vi "delay_image_analyseR2.vi"(0 "Image File List":string[](array[string])=["spectrum26270.000msh3000usd6.500dac0atoms.bny", "spectrum26270.000msh3000usd6.500dac1atoms.bny", "spectrum26270.000msh3000usd6.500dac2atoms.bny", "spectrum26270.000msh3000usd6.500dac3atoms.bny", "spectrum26270.000msh3000usd6.500dac4atoms.bny", "spectrum26270.000msh3000usd6.500dac5atoms.bny", "spectrum26270.000msh3000usd6.500dac6atoms.bny", "spectrum26270.000msh3000usd6.500dac7atoms.bny", "spectrum26270.000msh3000usd6.500dac8atoms.bny", "spectrum26270.000msh3000usd6.500dac9atoms.bny", "spectrum26270.000msh3000usd6.500dac10atoms.bny", "spectrum26270.000msh3000usd6.500dac11atoms.bny", "spectrum26270.000msh3000usd6.500dac12atoms.bny", "spectrum26270.000msh3000usd6.500dac13atoms.bny", "spectrum26270.000msh3000usd6.500dac14atoms.bny", "spectrum26270.000msh3000usd6.500dac15atoms.bny", "spectrum26270.000msh3000usd6.500dac16atoms.bny", "spectrum26270.000msh3000usd6.500dac17atoms.bny", "spectrum26270.000msh3000usd6.500dac18atoms.bny", "spectrum26270.000msh3000usd6.500dac19atoms.bny", "spectrum26270.000msh3000usd6.500dac20atoms.bny", "spectrum26270.000msh3000usd6.500dac21atoms.bny", "spectrum26270.000msh3000usd6.500dac22atoms.bny", "spectrum26270.000msh3000usd6.500dac23atoms.bny", "spectrum26270.000msh3000usd6.500dac24atoms.bny", "spectrum26270.000msh3000usd6.500dac25atoms.bny", "spectrum26270.000msh3000usd6.500dac26atoms.bny", "spectrum26270.000msh3000usd6.500dac27atoms.bny", "spectrum26270.000msh3000usd6.500dac28atoms.bny", "spectrum26270.000msh3000usd6.500dac29atoms.bny", "spectrum26270.000msh3000usd6.500dac30atoms.bny", "spectrum26270.000msh3000usd6.500dac31atoms.bny", "spectrum26270.000msh3000usd6.500dac32atoms.bny", "spectrum26270.000msh3000usd6.500dac33atoms.bny", "spectrum26270.000msh3000usd6.500dac34atoms.bny", "spectrum26270.000msh3000usd6.500dac35atoms.bny", "spectrum26270.000msh3000usd6.500dac36atoms.bny", "spectrum26270.000msh3000usd6.500dac37atoms.bny", "spectrum26270.000msh3000usd6.500dac38atoms.bny", "spectrum26270.000msh3000usd6.500dac39atoms.bny", "spectrum26270.000msh3000usd6.500dac40atoms.bny", "spectrum26270.000msh3000usd6.500dac41atoms.bny", "spectrum26270.000msh3000usd6.500dac42atoms.bny", "spectrum26270.000msh3000usd6.500dac43atoms.bny", "spectrum26270.000msh3000usd6.500dac44atoms.bny", "spectrum26270.000msh3000usd6.500dac45atoms.bny", "spectrum26270.000msh3000usd6.500dac46atoms.bny", "spectrum26270.000msh3000usd6.500dac47atoms.bny", "spectrum26270.000msh3000usd6.500dac48atoms.bny", "spectrum26270.000msh3000usd6.500dac49atoms.bny", "spectrum26270.000msh3000usd6.500dac50atoms.bny", "spectrum26270.000msh3000usd6.500dac51atoms.bny", "spectrum26270.000msh3000usd6.500dac52atoms.bny", "spectrum26270.000msh3000usd6.500dac53atoms.bny", "spectrum26270.000msh3000usd6.500dac54atoms.bny"], 1 "Background File List":string[](array[string])=["spectrum26270.000msh3000usd6.500dac0back.bny", "spectrum26270.000msh3000usd6.500dac1back.bny", "spectrum26270.000msh3000usd6.500dac2back.bny", "spectrum26270.000msh3000usd6.500dac3back.bny", "spectrum26270.000msh3000usd6.500dac4back.bny", "spectrum26270.000msh3000usd6.500dac5back.bny", "spectrum26270.000msh3000usd6.500dac6back.bny", "spectrum26270.000msh3000usd6.500dac7back.bny", "spectrum26270.000msh3000usd6.500dac8back.bny", "spectrum26270.000msh3000usd6.500dac9back.bny", "spectrum26270.000msh3000usd6.500dac10back.bny", "spectrum26270.000msh3000usd6.500dac11back.bny", "spectrum26270.000msh3000usd6.500dac12back.bny", "spectrum26270.000msh3000usd6.500dac13back.bny", "spectrum26270.000msh3000usd6.500dac14back.bny", "spectrum26270.000msh3000usd6.500dac15back.bny", "spectrum26270.000msh3000usd6.500dac16back.bny", "spectrum26270.000msh3000usd6.500dac17back.bny", "spectrum26270.000msh3000usd6.500dac18back.bny", "spectrum26270.000msh3000usd6.500dac19back.bny", "spectrum26270.000msh3000usd6.500dac20back.bny", "spectrum26270.000msh3000usd6.500dac21back.bny", "spectrum26270.000msh3000usd6.500dac22back.bny", "spectrum26270.000msh3000usd6.500dac23back.bny", "spectrum26270.000msh3000usd6.500dac24back.bny", "spectrum26270.000msh3000usd6.500dac25back.bny", "spectrum26270.000msh3000usd6.500dac26back.bny", "spectrum26270.000msh3000usd6.500dac27back.bny", "spectrum26270.000msh3000usd6.500dac28back.bny", "spectrum26270.000msh3000usd6.500dac29back.bny", "spectrum26270.000msh3000usd6.500dac30back.bny", "spectrum26270.000msh3000usd6.500dac31back.bny", "spectrum26270.000msh3000usd6.500dac32back.bny", "spectrum26270.000msh3000usd6.500dac33back.bny", "spectrum26270.000msh3000usd6.500dac34back.bny", "spectrum26270.000msh3000usd6.500dac35back.bny", "spectrum26270.000msh3000usd6.500dac36back.bny", "spectrum26270.000msh3000usd6.500dac37back.bny", "spectrum26270.000msh3000usd6.500dac38back.bny", "spectrum26270.000msh3000usd6.500dac39back.bny", "spectrum26270.000msh3000usd6.500dac40back.bny", "spectrum26270.000msh3000usd6.500dac41back.bny", "spectrum26270.000msh3000usd6.500dac42back.bny", "spectrum26270.000msh3000usd6.500dac43back.bny", "spectrum26270.000msh3000usd6.500dac44back.bny", "spectrum26270.000msh3000usd6.500dac45back.bny", "spectrum26270.000msh3000usd6.500dac46back.bny", "spectrum26270.000msh3000usd6.500dac47back.bny", "spectrum26270.000msh3000usd6.500dac48back.bny", "spectrum26270.000msh3000usd6.500dac49back.bny", "spectrum26270.000msh3000usd6.500dac50back.bny", "spectrum26270.000msh3000usd6.500dac51back.bny", "spectrum26270.000msh3000usd6.500dac52back.bny", "spectrum26270.000msh3000usd6.500dac53back.bny", "spectrum26270.000msh3000usd6.500dac54back.bny"], 3 "Image beam \nDetuning (MHz)":dbl=3.12 format="%.2f", 4 "Root Directory":path=path "C:/data/RedMOT/2007.01.10", 5 "Base Filename":string="coldMOT.04power4ms1645" caption="Base File Name (filename, base delay of column 10, and .dat will be added as extension.", 6 "scale base level?":bool, 7 "Natural Linewidth of Transition\n(ion fwhm in MHz)":dbl=32.0, 8 "Software Binning":T1={"Software\nBinning?"=TRUE, "Software Bin Size"=8}, 9 "Cut image?":bool, 10 "Wavelength (m)":dbl=4.61e-07, 11 "saved image dimensions":i32[](array[numeric])=[1024, 1280], 12 "Array of 6713\nValues":dbl[][](array[numeric])=[[6.5, 0.5, 0.04, 7.0, 1.75, 3.4, 3.8, 2.0], [6.5, 0.5, 0.04, 7.0, 1.75, 3.4, 3.8, 2.0], [6.5, 0.5, 0.04, 7.0, 1.75, 3.4, 3.8, 2.0], [6.5, 0.5, 0.04, 7.0, 1.75, 3.4, 3.8, 2.0], [6.5, 0.5, 0.04, 7.0, 1.75, 3.4, 3.8, 2.0], [6.5, 0.5, 0.04, 7.0, 1.75, 3.4, 3.8, 2.0], [6.5, 0.5, 0.04, 7.0, 1.75, 3.4, 3.8, 2.0], [6.5, 0.5, 0.04, 7.0, 1.75, 3.4, 3.8, 2.0], [6.5, 0.5, 0.04, 7.0, 1.75, 3.4, 3.8, 2.0], [6.5, 0.5, 0.04, 7.0, 1.75, 3.4, 3.8, 2.0], [6.5, 0.5, 0.04, 7.0, 1.75, 3.4, 3.8, 2.0], [6.5, 0.5, 0.04, 7.0, 1.75, 3.4, 3.8, 2.0], [6.5, 0.5, 0.04, 7.0, 1.75, 3.4, 3.8, 2.0], [6.5, 0.5, 0.04, 7.0, 1.75, 3.4, 3.8, 2.0], [6.5, 0.5, 0.04, 7.0, 1.75, 3.4, 3.8, 2.0], [6.5, 0.5, 0.04, 7.0, 1.75, 3.4, 3.8, 2.0], [6.5, 0.5, 0.04, 7.0, 1.75, 3.4, 3.8, 2.0], [6.5, 0.5, 0.04, 7.0, 1.75, 3.4, 3.8, 2.0], [6.5, 0.5, 0.04, 7.0, 1.75, 3.4, 3.8, 2.0], [6.5, 0.5, 0.04, 7.0, 1.75, 3.4, 3.8, 2.0], [6.5, 0.5, 0.04, 7.0, 1.75, 3.4, 3.8, 2.0], [6.5, 0.5, 0.04, 7.0, 1.75, 3.4, 3.8, 2.0], [6.5, 0.5, 0.04, 7.0, 1.75, 3.4, 3.8, 2.0], [6.5, 0.5, 0.04, 7.0, 1.75, 3.4, 3.8, 2.0], [6.5, 0.5, 0.04, 7.0, 1.75, 3.4, 3.8, 2.0], [6.5, 0.5, 0.04, 7.0, 1.75, 3.4, 3.8, 2.0], [6.5, 0.5, 0.04, 7.0, 1.75, 3.4, 3.8, 2.0], [6.5, 0.5, 0.04, 7.0, 1.75, 3.4, 3.8, 2.0], [6.5, 0.5, 0.04, 7.0, 1.75, 3.4, 3.8, 2.0], [6.5, 0.5, 0.04, 7.0, 1.75, 3.4, 3.8, 2.0], [6.5, 0.5, 0.04, 7.0, 1.75, 3.4, 3.8, 2.0], [6.5, 0.5, 0.04, 7.0, 1.75, 3.4, 3.8, 2.0], [6.5, 0.5, 0.04, 7.0, 1.75, 3.4, 3.8, 2.0], [6.5, 0.5, 0.04, 7.0, 1.75, 3.4, 3.8, 2.0], [6.5, 0.5, 0.04, 7.0, 1.75, 3.4, 3.8, 2.0], [6.5, 0.5, 0.04, 7.0, 1.75, 3.4, 3.8, 2.0], [6.5, 0.5, 0.04, 7.0, 1.75, 3.4, 3.8, 2.0], [6.5, 0.5, 0.04, 7.0, 1.75, 3.4, 3.8, 2.0], [6.5, 0.5, 0.04, 7.0, 1.75, 3.4, 3.8, 2.0], [6.5, 0.5, 0.04, 7.0, 1.75, 3.4, 3.8, 2.0], [6.5, 0.5, 0.04, 7.0, 1.75, 3.4, 3.8, 2.0], [6.5, 0.5, 0.04, 7.0, 1.75, 3.4, 3.8, 2.0], [6.5, 0.5, 0.04, 7.0, 1.75, 3.4, 3.8, 2.0], [6.5, 0.5, 0.04, 7.0, 1.75, 3.4, 3.8, 2.0], [6.5, 0.5, 0.04, 7.0, 1.75, 3.4, 3.8, 2.0], [6.5, 0.5, 0.04, 7.0, 1.75, 3.4, 3.8, 2.0], [6.5, 0.5, 0.04, 7.0, 1.75, 3.4, 3.8, 2.0], [6.5, 0.5, 0.04, 7.0, 1.75, 3.4, 3.8, 2.0], [6.5, 0.5, 0.04, 7.0, 1.75, 3.4, 3.8, 2.0], [6.5, 0.5, 0.04, 7.0, 1.75, 3.4, 3.8, 2.0], [6.5, 0.5, 0.04, 7.0, 1.75, 3.4, 3.8, 2.0], [6.5, 0.5, 0.04, 7.0, 1.75, 3.4, 3.8, 2.0], [6.5, 0.5, 0.04, 7.0, 1.75, 3.4, 3.8, 2.0], [6.5, 0.5, 0.04, 7.0, 1.75, 3.4, 3.8, 2.0], [6.5, 0.5, 0.04, 7.0, 1.75, 3.4, 3.8, 2.0]], 13 "ROI Controls":T5={"col index"=400, "col length"=700, "row index"=800, "row length"=100}, 14 "Specifics of Fitting Routines":T4={"sampleinterleave"=1.0, "pixelsize"=1.04e-05, "CCD Binning"=1.0, "cutborders"=0.0, "numberforscale"=5.0, "limit"=5.0, "guesssmoothsize"=1.0}, 15 "Changed\nValue":dbl[](array[numeric])=[163.9, 163.95000000000002, 164.00000000000003, 164.05000000000004, 164.10000000000005, 164.15000000000006, 164.20000000000007, 164.25000000000009, 164.3000000000001, 164.3500000000001, 164.40000000000012, 164.45000000000013, 164.50000000000014, 164.55000000000015, 164.60000000000016, 164.65000000000018, 164.7000000000002, 164.7500000000002, 164.8000000000002, 164.85000000000022, 164.90000000000023, 164.95000000000024, 165.00000000000026, 165.05000000000027, 165.10000000000028, 165.1500000000003, 165.2000000000003, 165.2500000000003, 165.30000000000032, 165.35000000000034, 165.40000000000035, 165.45000000000036, 165.50000000000037, 165.55000000000038, 165.6000000000004, 165.6500000000004, 165.70000000000041, 165.75000000000043, 165.80000000000044, 165.85000000000045, 165.90000000000046, 165.95000000000047, 166.00000000000048, 166.0500000000005, 166.1000000000005, 166.15000000000052, 166.20000000000053, 166.25000000000054, 166.30000000000055, 166.35000000000056, 166.40000000000057, 166.45000000000059, 166.5000000000006, 166.5500000000006, 166.60000000000062], 17 "Load File Names\nFrom Batch File?":bool, 18 "fmot":dbl=-86.7, 19 "camera background with no image beam\nIt will be subtracted before the log is taken":i8) -> ()   [LabVIEW 2013]
uses:
  <vilib>/Analysis/NI_AALPro.lvlib
  <vilib>/Utility/file.llb/Read From Spreadsheet File (DBL).vi
panel:
  in  "Read\nBinary?":bool=TRUE
  out "Iteration Number":i32=9
  in  "Overwrite existing image.fit files on \nstand-alone delayimageanalyse run?":bool
  out "Background File List":string[](array[string])=["coldMOT.04power4ms16450.000msh300usd6.500dac0back.bny", "coldMOT.04power4ms16450.000msh600usd6.500dac1back.bny", "coldMOT.04power4ms16450.000msh899usd6.500dac2back.bny", "coldMOT.04power4ms16450.000msh1200usd6.500dac3back.bny", "coldMOT.04power4ms16450.000msh1500usd6.500dac4back.bny", "coldMOT.04power4ms16450.000msh1800usd6.500dac5back.bny", "coldMOT.04power4ms16450.000msh2100usd6.500dac6back.bny", "coldMOT.04power4ms16450.000msh2400usd6.500dac7back.bny", "coldMOT.04power4ms16450.000msh2699usd6.500dac8back.bny", "coldMOT.04power4ms16450.000msh2999usd6.500dac9back.bny"]
  out "Image File List":string[](array[string])=["coldMOT.04power4ms16450.000msh300usd6.500dac0atoms.bny", "coldMOT.04power4ms16450.000msh600usd6.500dac1atoms.bny", "coldMOT.04power4ms16450.000msh899usd6.500dac2atoms.bny", "coldMOT.04power4ms16450.000msh1200usd6.500dac3atoms.bny", "coldMOT.04power4ms16450.000msh1500usd6.500dac4atoms.bny", "coldMOT.04power4ms16450.000msh1800usd6.500dac5atoms.bny", "coldMOT.04power4ms16450.000msh2100usd6.500dac6atoms.bny", "coldMOT.04power4ms16450.000msh2400usd6.500dac7atoms.bny", "coldMOT.04power4ms16450.000msh2699usd6.500dac8atoms.bny", "coldMOT.04power4ms16450.000msh2999usd6.500dac9atoms.bny"]
  in  "Tab Control 2":enum32{"Fit Values"}(tab)
  out "2D fits":T2(array[cluster])=[{"amplitude"=0.5738165225547651, "sigma_x (m)"=0.001779968905776355, "sigma_y (m)"=0.0017979290921732018, "x offset"=27.55112062319906, "y offset"=14.91641160525659, "offset"=0.015742195394534482, "slope x"=0.00014578412333354483, "slope y"=-0.00022622923779412406, 0.0}, {"amplitude"=0.5281671733235853, "sigma_x (m)"=0.0018356867534323564, "sigma_y (m)"=0.0018447422111293492, "x offset"=27.475051790813755, "y offset"=14.884754628668023, "offset"=-0.003445615025672064, "slope x"=2.120808325107998e-05, "slope y"=0.00017802536724854167, 0.0}, {"amplitude"=0.5064742768085322, "sigma_x (m)"=0.0018698692022573722, "sigma_y (m)"=0.0018794073643444349, "x offset"=27.428973678087967, "y offset"=14.847963381339092, "offset"=0.002951397507155775, "slope x"=1.9051434324983357e-06, "slope y"=0.0002301898004673639, 0.0}, {"amplitude"=0.4797175377868185, "sigma_x (m)"=0.0019159519765526297, "sigma_y (m)"=0.0019326008236855527, "x offset"=27.25509949811987, "y offset"=14.842720250554702, "offset"=-0.0027884361829993713, "slope x"=1.151258895737645e-05, "slope y"=0.0002143184116028636, 0.0}, {"amplitude"=0.461485871518208, "sigma_x (m)"=0.0019474973318284335, "sigma_y (m)"=0.0019711563089907748, "x offset"=27.210211909744878, "y offset"=14.769209555472836, "offset"=-0.0026707277113455856, "slope x"=1.5808562999497198e-06, "slope y"=0.00019245433859413762, 0.0}, {"amplitude"=0.4337958365249558, "sigma_x (m)"=0.0019988093267557312, "sigma_y (m)"=0.0020227446205385857, "x offset"=27.151306462350345, "y offset"=14.748046257715934, "offset"=0.0018997667357263921, "slope x"=1.0845989105090682e-05, "slope y"=0.0001669337070974055, 0.0}, {"amplitude"=0.4181668162660838, "sigma_x (m)"=0.0020407468762672675, "sigma_y (m)"=0.002072739235917522, "x offset"=27.063234090928052, "y offset"=14.7573800473226, "offset"=-0.004199802256870902, "slope x"=1.762210333484681e-05, "slope y"=0.0001323033741165302, 0.0}, {"amplitude"=0.39682375154213595, "sigma_x (m)"=0.0021117452562746304, "sigma_y (m)"=0.002150734064213093, "x offset"=26.994041203086788, "y offset"=14.7356469057076, "offset"=2.7036082185703935e-06, "slope x"=2.3077172179815774e-05, "slope y"=0.00013946938043275634, 0.0}, {"amplitude"=0.3680872238335552, "sigma_x (m)"=0.0021637337440412025, "sigma_y (m)"=0.002228488332265176, "x offset"=26.87934998105081, "y offset"=14.613638917171995, "offset"=0.00243715359412698, "slope x"=3.29653335875719e-05, "slope y"=0.0001222395516569478, 0.0}, {"amplitude"=0.34737870644503205, "sigma_x (m)"=0.002225541779498022, "sigma_y (m)"=0.002301338517452132, "x offset"=26.840946026057907, "y offset"=14.670687821740248, "offset"=-0.0008286207749249162, "slope x"=4.498190646953117e-05, "slope y"=8.518232221332428e-05, 0.0}]
  out "1D fits":T3(array[cluster])=[{"Numeric"=0.3, "Amplitude"=7.504466228512422, "rmswidthx"=0.00014339243450146302, "offsetx"=5.5169543980856765e-05, "numberx"=0.684674611713356, "Amplitude"=110353.68163127101, "y0"=7.90148216419731, "rmswidthy"=0.00027667492426750056, "offsety"=5.640246639784781e-05, "numbery"=0.3704720097868406, "alpha"=118788.46888827615, "peakdensity"=9.780378189411328e-14, 4.1613004340832936e+16, "number"=0.5628258585929871, 112511.20036655785, 0.0, 0.0, 0.0, "x0"=0.0}, {"Numeric"=0.6, "Amplitude"=6.956785475959535, "rmswidthx"=0.00014503490220851433, "offsetx"=5.4426146748675424e-05, "numberx"=0.15035610250846762, "Amplitude"=100921.52970869098, "y0"=7.421767741978517, "rmswidthy"=0.0002754321721409688, "offsety"=5.786695612483155e-05, "numbery"=-0.16868185571059519, "alpha"=114473.67433086078, "peakdensity"=9.780378189411328e-14, 3.741980093960017e+16, "number"=0.4992920458316803, 101022.26245184144, 0.0, 0.0, 0.0, "x0"=0.0}, {"Numeric"=0.9, "Amplitude"=6.75653556442615, "rmswidthx"=0.0001449283703698668, "offsetx"=5.52095402934212e-05, "numberx"=0.43775356220056916, "Amplitude"=99427.3405179374, "y0"=7.233315694451832, "rmswidthy"=0.0002748899433133735, "offsety"=5.9025951942169804e-05, "numbery"=0.044148021940494525, "alpha"=113801.5153292087, "peakdensity"=9.780378189411328e-14, 3.5954506885908052e+16, "number"=0.4866458773612976, 101881.28200144663, 0.0, 0.0, 0.0, "x0"=0.0}, {"Numeric"=1.2, "Amplitude"=6.522468405836582, "rmswidthx"=0.00014489042466375092, "offsetx"=5.6659883530226195e-05, "numberx"=0.21993088671427027, "Amplitude"=98504.32209359134, "y0"=7.035558997618763, "rmswidthy"=0.000273285078777017, "offsety"=6.062554611589187e-05, "numbery"=-0.14787126367796644, "alpha"=113689.90353099872, "peakdensity"=9.780378189411328e-14, 3.2911491986496572e+16, "number"=0.4571606516838074, 100884.48746492954, 0.0, 0.0, 0.0, "x0"=0.0}, {"Numeric"=1.5, "Amplitude"=6.362746658409087, "rmswidthx"=0.00014396081252980266, "offsetx"=5.780955638880978e-05, "numberx"=0.22689293011073247, "Amplitude"=98041.93933259645, "y0"=6.885127347526461, "rmswidthy"=0.0002727848778688392, "offsety"=6.161710048792166e-05, "numbery"=-0.13900329269281128, "alpha"=113078.7138670004, "peakdensity"=9.780378189411328e-14, 3.0969773037552796e+16, "number"=0.4389178454875946, 100440.38218616454, 0.0, 0.0, 0.0, "x0"=0.0}, {"Numeric"=1.8, "Amplitude"=6.119823356085586, "rmswidthx"=0.00014361802341762025, "offsetx"=5.925492272334584e-05, "numberx"=0.4067212745742367, "Amplitude"=96656.47392619436, "y0"=6.631385347864259, "rmswidthy"=0.00027218984808309777, "offsety"=6.330358795367532e-05, "numbery"=0.0017852093930514896, "alpha"=111892.3039087028, "peakdensity"=9.780378189411328e-14, 2.88164856532834e+16, "number"=0.4186113774776459, 100876.0377296957, 0.0, 0.0, 0.0, "x0"=0.0}, {"Numeric"=2.1, "Amplitude"=6.017825904261809, "rmswidthx"=0.0001434953763372387, "offsetx"=6.0780011507120856e-05, "numberx"=0.15558716442749868, "Amplitude"=97491.78507550228, "y0"=6.537153639451476, "rmswidthy"=0.00027134483402538946, "offsety"=6.468245180449752e-05, "numbery"=-0.19848806955625203, "alpha"=112704.89809609308, "peakdensity"=9.780378189411328e-14, 2.680044464213022e+16, "number"=0.3993450999259949, 100860.20149904813, 0.0, 0.0, 0.0, "x0"=0.0}, {"Numeric"=2.4, "Amplitude"=5.873872189954546, "rmswidthx"=0.00014344834753399392, "offsetx"=6.28251076220572e-05, "numberx"=0.3436470260174619, "Amplitude"=98361.54883252039, "y0"=6.41233299233666, "rmswidthy"=0.0002706321856826436, "offsety"=6.692710223497914e-05, "numbery"=-0.0643190721262936, "alpha"=114389.38202594258, "peakdensity"=9.780378189411328e-14, 2.502093511768087e+16, "number"=0.38537395000457764, 104097.8700150471, 0.0, 0.0, 0.0, "x0"=0.0}, {"Numeric"=2.7, "Amplitude"=5.568117736893174, "rmswidthx"=0.00014206501901669244, "offsetx"=6.513858863664371e-05, "numberx"=0.42899869366090154, "Amplitude"=96675.04417787395, "y0"=6.133188707922994, "rmswidthy"=0.0002696058226529639, "offsety"=6.855331269383554e-05, "numbery"=0.01443494853680136, "alpha"=112068.20048635374, "peakdensity"=9.780378189411328e-14, 2.252616266610856e+16, "number"=0.3597254455089569, 103195.8311672371, 0.0, 0.0, 0.0, "x0"=0.0}, {"Numeric"=3.0, "Amplitude"=5.393804464980791, "rmswidthx"=0.0001424497022558477, "offsetx"=6.737453651540354e-05, "numberx"=0.2834182795584339, "Amplitude"=96863.15575321819, "y0"=5.956695315529496, "rmswidthy"=0.000269292839928873, "offsety"=7.054634826962447e-05, "numbery"=-0.0963891836808563, "alpha"=112007.6149375534, "peakdensity"=9.780378189411328e-14, 2.042331084856188e+16, "number"=0.33733975887298584, 103005.8924570147, 0.0, 0.0, 0.0, "x0"=0.0}] {"x0" format="%.2f"; "?" format="%.2f"; "?" format="%.2f"; "?" format="%.2f"; "?" format="%.2e"; "?" format="%.2e"; "number" format="%.2e"; "peakdensity" format="%.2e"; "alpha" format="%.2e"; "numbery" format="%.2e"; "offsety" format="%.2e"; "rmswidthy" format="%.2e"; "y0" format="%.2e"; "Amplitude" format="%.2e"; "numberx" format="%.2f"; "offsetx" format="%.2e"; "rmswidthx" format="%.2e"; "Amplitude" format="%.2e"; "Numeric" format="%.2f"}
  in  "Tab Control":enum32{"Fits"}(tab)
  out "Peak OD versus delay":cluster{dbl[], dbl[]}(graph)={[0.3, 0.6, 0.9, 1.2, 1.5, 1.8, 2.1, 2.4, 2.7, 3.0], [0.5738165225547651, 0.5281671733235853, 0.5064742768085322, 0.4797175377868185, 0.461485871518208, 0.4337958365249558, 0.4181668162660838, 0.39682375154213595, 0.3680872238335552, 0.34737870644503205]}
  out "Temperature (mK) x":dbl=2.367635340521096 format="%.7f"
  out "Mean Square\nError x 2D Fit":dbl=5.270568634913362e-08 format="%.2e"
  out "Initial Size x 2D Fit":dbl=0.001826492989267636 format="%.2e"
  out "Temperature (mK) y":dbl=2.0156813164871936 format="%.7f"
  out "Mean Square \nError y 2D Fit":dbl=7.02341970388832e-08 format="%.2e"
  out "Initial Size y 2D Fit":dbl=0.001821925810077018 format="%.2e"
  out "RMS Width X 2D Fit":cluster{"Changed\nValue":dbl[], dbl[]}[](graph)=[{"Changed\nValue"=[0.3, 0.6, 0.9, 1.2, 1.5, 1.8, 2.1, 2.4, 2.7, 3.0], [0.0017979290921732018, 0.0018447422111293492, 0.0018794073643444349, 0.0019326008236855527, 0.0019711563089907748, 0.0020227446205385857, 0.002072739235917522, 0.002150734064213093, 0.002228488332265176, 0.002301338517452132]}, {"Changed\nValue"=[0.3, 0.6, 0.9, 1.2, 1.5, 1.8, 2.1, 2.4, 2.7, 3.0], [0.001831962015386798, 0.0018482719993953172, 0.0018751400784021274, 0.0019121212345098776, 0.001958642716079094, 0.00201404352857337, 0.002077613475283437, 0.0021486275950761777, 0.0022263736667322556, 0.0023101721229093052]}]
  out "RMS Width Y 2D Fit":cluster{"Changed\nValue":dbl[], dbl[]}[](graph)=[{"Changed\nValue"=[0.3, 0.6, 0.9, 1.2, 1.5, 1.8, 2.1, 2.4, 2.7, 3.0], [0.001779968905776355, 0.0018356867534323564, 0.0018698692022573722, 0.0019159519765526297, 0.0019474973318284335, 0.0019988093267557312, 0.0020407468762672675, 0.0021117452562746304, 0.0021637337440412025, 0.002225541779498022]}, {"Changed\nValue"=[0.3, 0.6, 0.9, 1.2, 1.5, 1.8, 2.1, 2.4, 2.7, 3.0], [0.0018265945319208092, 0.0018405296422219352, 0.001863523275140027, 0.0018952457580261259, 0.0019352678943443048, 0.0019830872435876484, 0.002038155063216898, 0.0020999011788628776, 0.0021677549938817187, 0.002241161823529252]}]
  out "RMS Widths Graph":cluster{"Delay (usec)":dbl[], dbl[]}[](graph)=[{"Delay (usec)"=[0.3, 0.6, 0.9, 1.2, 1.5, 1.8, 2.1, 2.4, 2.7, 3.0], [0.0017979290921732018, 0.0018447422111293492, 0.0018794073643444349, 0.0019326008236855527, 0.0019711563089907748, 0.0020227446205385857, 0.002072739235917522, 0.002150734064213093, 0.002228488332265176, 0.002301338517452132]}, {"Delay (usec)"=[0.3, 0.6, 0.9, 1.2, 1.5, 1.8, 2.1, 2.4, 2.7, 3.0], [0.001779968905776355, 0.0018356867534323564, 0.0018698692022573722, 0.0019159519765526297, 0.0019474973318284335, 0.0019988093267557312, 0.0020407468762672675, 0.0021117452562746304, 0.0021637337440412025, 0.002225541779498022]}]
  out "Number Graph":cluster{"Delay (usec)":dbl[], dbl[]}(graph)={"Delay (usec)"=[0.3, 0.6, 0.9, 1.2, 1.5, 1.8, 2.1, 2.4, 2.7, 3.0], [118779709.2973507, 112397163.6012744, 111223499.04059331, 110893006.78441514, 110405764.53942999, 109109669.88416144, 109946506.4260554, 111346428.37145746, 109132043.66837342, 108972793.36629671]}
  out "sqrt(KT/M) Y":dbl=0.013885336188842719 format="%.2e"
  out "initial size x":dbl=5.4258675810882964e-05 format="%.2e"
  out "sqrt(KT/M) x":dbl=0.013269260868114613 format="%.2e"
  out "Temperature (mK) X":dbl=0.0018751804744517283 format="%.7f"
  out "Temperature (mK) Y":dbl=0.002053347275472023 format="%.7f"
  out "initial size Y":dbl=5.757790007542504e-05 format="%.2e"
  out "RMS width fity":cluster{"Changed\nValue":dbl[], dbl[]}[](graph)=[{"Changed\nValue"=[0.3, 0.6, 0.9, 1.2, 1.5, 1.8, 2.1, 2.4, 2.7, 3.0], [5.7728388229644674e-05, 5.817751712718082e-05, 5.891845764756704e-05, 5.994038926339049e-05, 6.122924415276819e-05, 6.276858190994688e-05, 6.45404824234063e-05, 6.652636566730681e-05, 6.870767968246571e-05, 7.106643108240556e-05]}, {"Changed\nValue"=[0.3, 0.6, 0.9, 1.2, 1.5, 1.8, 2.1, 2.4, 2.7, 3.0], [5.640246639784781e-05, 5.786695612483155e-05, 5.9025951942169804e-05, 6.062554611589187e-05, 6.161710048792166e-05, 6.330358795367532e-05, 6.468245180449752e-05, 6.692710223497914e-05, 6.855331269383554e-05, 7.054634826962447e-05]}]
  out "RMS width fitx":cluster{"Changed\nValue":dbl[], dbl[]}[](graph)=[{"Changed\nValue"=[0.3, 0.6, 0.9, 1.2, 1.5, 1.8, 2.1, 2.4, 2.7, 3.0], [5.440450805134849e-05, 5.4839677998557614e-05, 5.555738709459993e-05, 5.65468781604294e-05, 5.779419339102477e-05, 5.928306116307919e-05, 6.099579561846127e-05, 6.291411619430335e-05, 6.501982882943482e-05, 6.729534498481448e-05]}, {"Changed\nValue"=[0.3, 0.6, 0.9, 1.2, 1.5, 1.8, 2.1, 2.4, 2.7, 3.0], [5.5169543980856765e-05, 5.4426146748675424e-05, 5.52095402934212e-05, 5.6659883530226195e-05, 5.780955638880978e-05, 5.925492272334584e-05, 6.0780011507120856e-05, 6.28251076220572e-05, 6.513858863664371e-05, 6.737453651540354e-05]}]
  out "Number":cluster{"Delay (usec)":dbl[], dbl[]}[](graph)=[{"Delay (usec)"=[0.3, 0.6, 0.9, 1.2, 1.5, 1.8, 2.1, 2.4, 2.7, 3.0], [110353.68163127101, 100921.52970869098, 99427.3405179374, 98504.32209359134, 98041.93933259645, 96656.47392619436, 97491.78507550228, 98361.54883252039, 96675.04417787395, 96863.15575321819]}, {"Delay (usec)"=[0.3, 0.6, 0.9, 1.2, 1.5, 1.8, 2.1, 2.4, 2.7, 3.0], [118788.46888827615, 114473.67433086078, 113801.5153292087, 113689.90353099872, 113078.7138670004, 111892.3039087028, 112704.89809609308, 114389.38202594258, 112068.20048635374, 112007.6149375534]}]
  out "RMS width":cluster{"Delay (usec)":dbl[], dbl[]}[](graph)=[{"Delay (usec)"=[0.3, 0.6, 0.9, 1.2, 1.5, 1.8, 2.1, 2.4, 2.7, 3.0], [5.5169543980856765e-05, 5.4426146748675424e-05, 5.52095402934212e-05, 5.6659883530226195e-05, 5.780955638880978e-05, 5.925492272334584e-05, 6.0780011507120856e-05, 6.28251076220572e-05, 6.513858863664371e-05, 6.737453651540354e-05]}, {"Delay (usec)"=[0.3, 0.6, 0.9, 1.2, 1.5, 1.8, 2.1, 2.4, 2.7, 3.0], [5.640246639784781e-05, 5.786695612483155e-05, 5.9025951942169804e-05, 6.062554611589187e-05, 6.161710048792166e-05, 6.330358795367532e-05, 6.468245180449752e-05, 6.692710223497914e-05, 6.855331269383554e-05, 7.054634826962447e-05]}]
  in  "1D fits?":bool=TRUE
  out "mean square error":dbl=4.707333442670224e-21 format="%.2e"
  # "These lists only change\nwhen input is from PB."
  # "Controls"
  # "If so, you only need to input the root directory and the base file name."
  # "These are only indicators of file list."
  # "Sigma^2=(sigma_0)^2+(KT/M)t^2"
  # "2D Fit Values"
  # "1D Fit Values"
  # "(total column size in each data file should be an integer multiple of sampleinterleave) for big matrices form a matrix using only one point for every sampleinterleave points in a row/column"
  # "number of columns and rows to scale the base level of atom and background images"
  # "the real size for the object in meter unit for a pixel"
  # "number of columns and rows at the corners to find the uncertainties/noise"
  # "total binning"
  # "(REMEMBER THIS IS DONE AFTER SAMPLEINTERLEAVE) number of columns and rows to trim on either side of the data matrix"
  # "number of pixels in smoothing for plotting residuals"
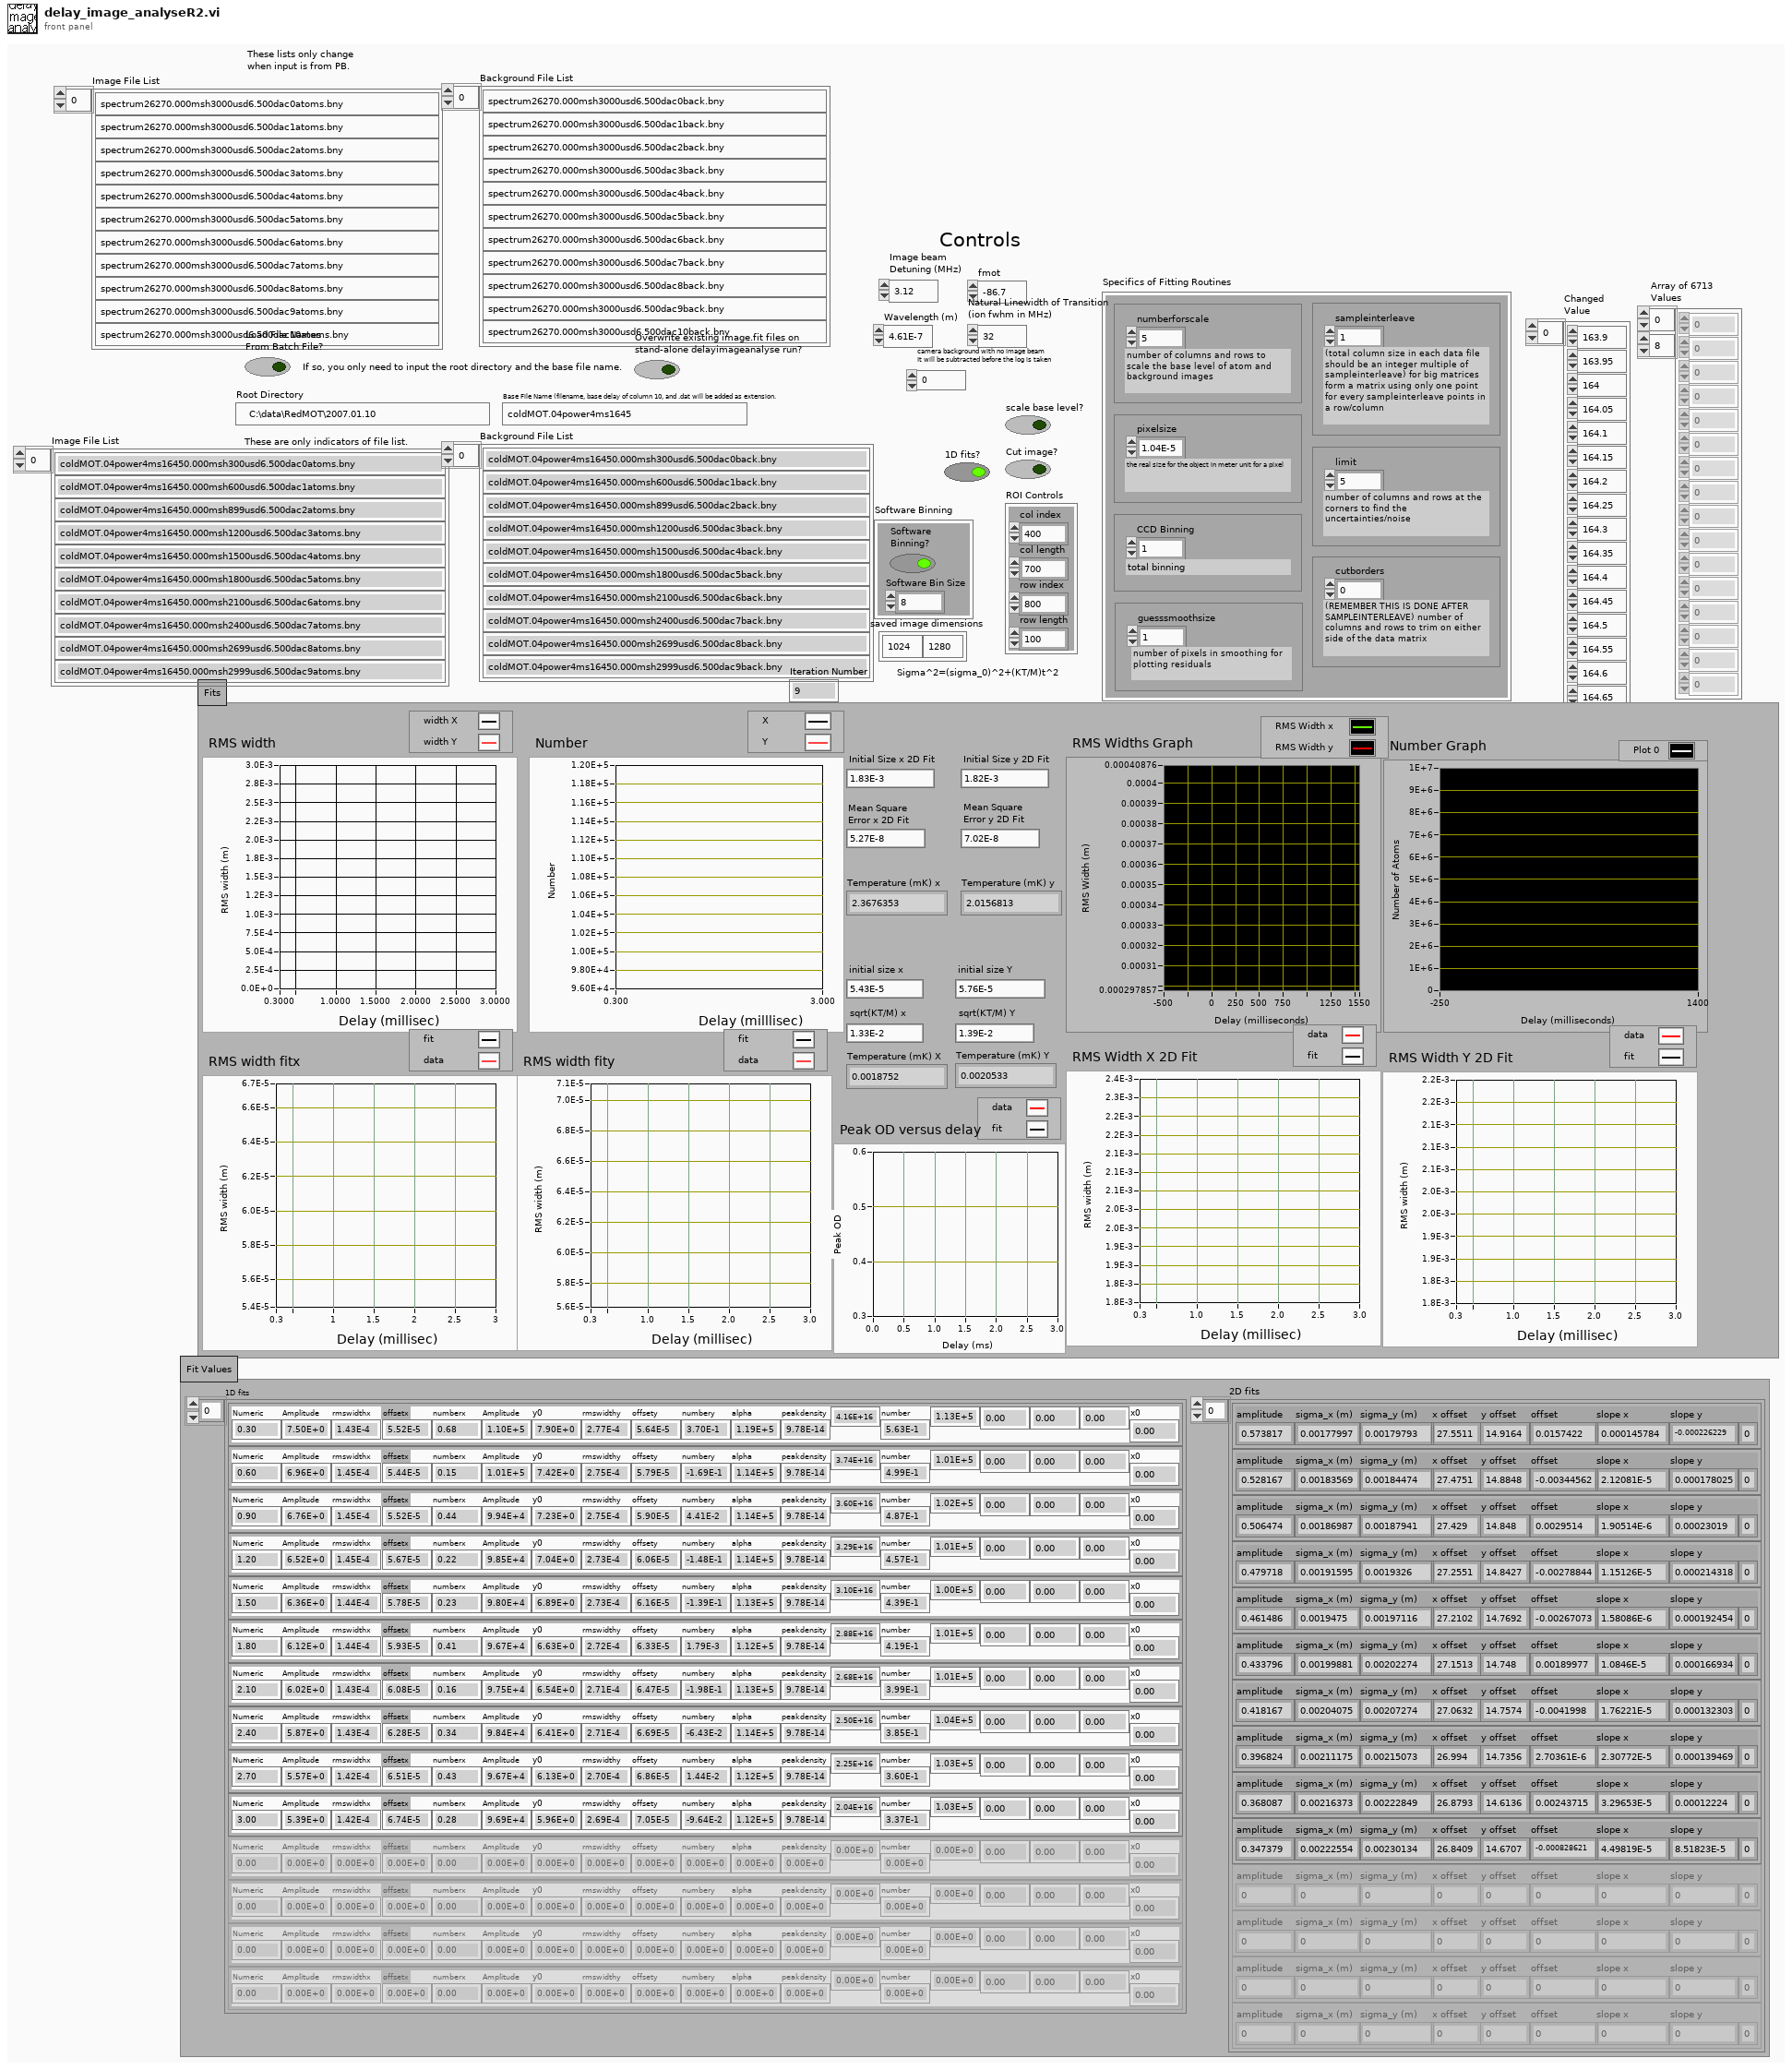
[diagram p1: front panel]
types:
  T1 = cluster{"Software\nBinning?":bool, "Software Bin Size":i32}
  T2 = cluster{"amplitude":dbl, "sigma_x (m)":dbl, "sigma_y (m)":dbl, "x offset":dbl, "y offset":dbl, "offset":dbl, "slope x":dbl, "slope y":dbl, dbl}[]
  T3 = cluster{"Numeric":dbl, "Amplitude":dbl, "rmswidthx":dbl, "offsetx":dbl, "numberx":dbl, "Amplitude":dbl, "y0":dbl, "rmswidthy":dbl, "offsety":dbl, "numbery":dbl, "alpha":dbl, "peakdensity":dbl, dbl, "number":dbl, dbl, dbl, dbl, dbl, "x0":dbl}[]
  T4 = cluster{"sampleinterleave":dbl, "pixelsize":dbl, "CCD Binning":dbl, "cutborders":dbl, "numberforscale":dbl, "limit":dbl, "guesssmoothsize":dbl}
  T5 = cluster{"col index":i32, "col length":i32, "row index":i32, "row length":i32}
  T6 = cluster{"amplitude":dbl, "sigma_y (m)":dbl, "sigma_x (m)":dbl, "row offset (pixel #)":dbl, "col offset (pixel #)":dbl, "offset":dbl, "slope x":dbl, "slope y":dbl, dbl}
  T7 = cluster{"Amplitude":dbl, "x0":dbl, "rmswidthx":dbl, "offsetx":dbl, "numberx":dbl}
  T8 = cluster{"alpha":dbl, "peakdensity":dbl, "alphadenssigzsqrt2pi":sgl, "number":dbl}
  T9 = cluster{"Amplitude":dbl, "y0":dbl, "rmswidthy":dbl, "offsety":dbl, "numbery":dbl}
  T10 = cluster{"Wavelength (m)":dbl, "Natural Linewidth of Transition\n(ion fwhm in MHz)":dbl, "Image beam \nDetuning (MHz)":dbl, "sampleinterleave":dbl, "pixelsize":dbl, "cutborders":dbl, "numberforscale":dbl, "limit":dbl, "guesssmoothsize":dbl, "amplitude":dbl, "sigma_y (m)":dbl, "sigma_x (m)":dbl, "row offset (pixel #)":dbl, "col offset (pixel #)":dbl, "offset":dbl, "slope x":dbl, "slope y":dbl, "Chi-squared":dbl, "# atoms from peakOD":dbl}
  T11 = cluster{"Numeric":dbl, "Amplitude":dbl, "x0":dbl, "rmswidthx":dbl, "offsetx":dbl, "numberx":dbl, "Amplitude":dbl, "y0":dbl, "rmswidthy":dbl, "offsety":dbl, "numbery":dbl, "alpha":dbl, "peakdensity":dbl, dbl, "number":dbl, dbl, dbl, dbl, dbl}
  T12 = cluster{"Array of 6713\nValues[0]":dbl, "Array of 6713\nValues[1]":dbl, "Array of 6713\nValues[2]":dbl, "Array of 6713\nValues[3]":dbl, "Array of 6713\nValues[4]":dbl, "Array of 6713\nValues[5]":dbl, "Array of 6713\nValues[6]":dbl, "Array of 6713\nValues[7]":dbl, "Array of 6713\nValues[8]":dbl}
  T13 = cluster{"fmot":dbl, "Array of 6713\nValues[0]":dbl, "Array of 6713\nValues[1]":dbl, "Array of 6713\nValues[2]":dbl, "Array of 6713\nValues[3]":dbl, "Array of 6713\nValues[4]":dbl, "Array of 6713\nValues[5]":dbl, "Array of 6713\nValues[6]":dbl, "Array of 6713\nValues[8]":dbl, "Numeric":dbl, "Amplitude":dbl, "x0":dbl, "rmswidthx":dbl, "offsetx":dbl, "numberx":dbl, "Amplitude":dbl, "y0":dbl, "rmswidthy":dbl, "offsety":dbl, "numbery":dbl, "alpha":dbl, "peakdensity":dbl, dbl, "number":dbl}
  T14 = cluster{"Array of 6713\nValues[0]":dbl, "Array of 6713\nValues[1]":dbl, "Array of 6713\nValues[2]":dbl, "Array of 6713\nValues[3]":dbl, "Array of 6713\nValues[4]":dbl, "Array of 6713\nValues[5]":dbl, "Array of 6713\nValues[6]":dbl, "Array of 6713\nValues[7]":dbl, "Array of 6713\nValues[8]":dbl, "Wavelength (m)":dbl, "Natural Linewidth of Transition\n(ion fwhm in MHz)":dbl, "Image beam \nDetuning (MHz)":dbl, "sampleinterleave":dbl, "pixelsize":dbl, "cutborders":dbl, "numberforscale":dbl, "limit":dbl, "guesssmoothsize":dbl, "amplitude":dbl, "sigma_y (m)":dbl, "sigma_x (m)":dbl, "row offset (pixel #)":dbl, "col offset (pixel #)":dbl, "offset":dbl, "slope x":dbl, "slope y":dbl, "Chi-squared":dbl, "# atoms from peakOD":dbl}
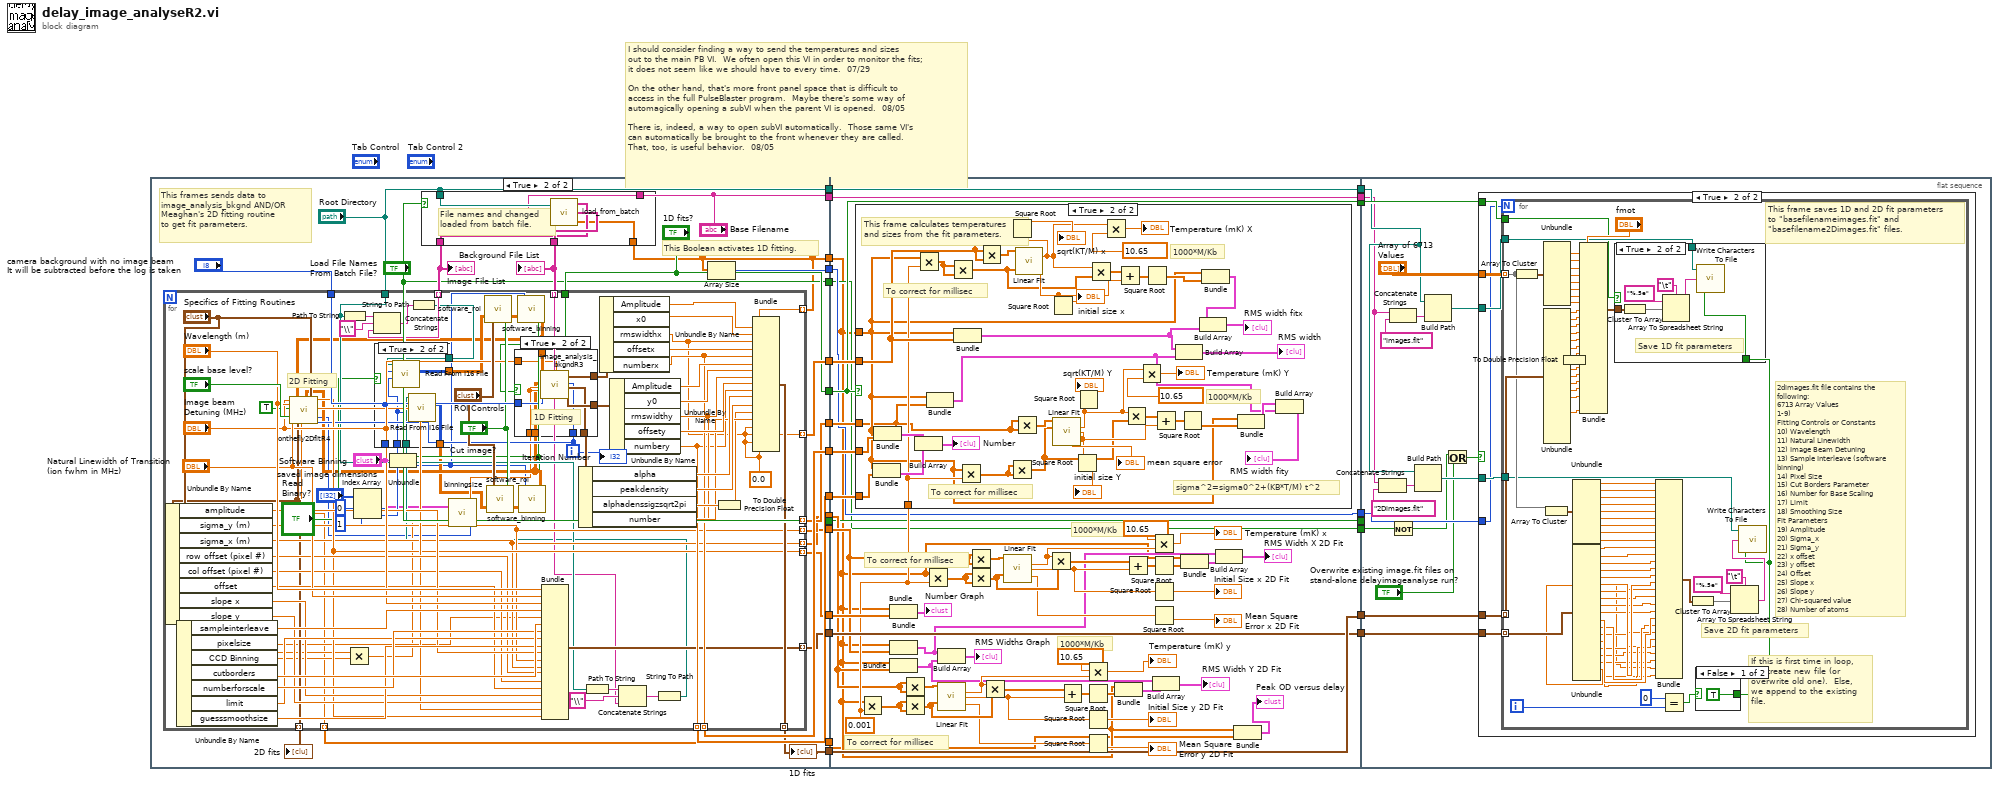
[diagram p0: block diagram]
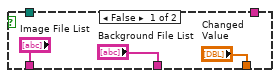
[diagram p2: hidden frame]
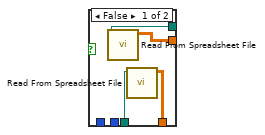
[diagram p3: hidden frame]
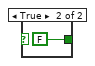
[diagram p7: hidden frame]
diagram:
  # "I should consider finding a way to send the temperatures and sizes\nout to the main PB VI.  We often open this VI in order to monitor the fits;\nit does not seem like we should have to every time.  07/29\n\nOn the other hand, that's more front panel space that is difficult to\naccess in the full PulseBlaster program.  Maybe there's some way of\nautomagically opening a subVI when the parent VI is opened.  08/05\n\nThere is, indeed, a way to open subVI automatically.  Those same VI's\ncan automatically be brought to the front whenever they are called.\nThat, too, is useful behavior.  08/05"
  n1 = flat-sequence {
    tunnel: [w27] -> w25
    tunnel: [w44] -> w24
    tunnel: [w43] -> w23
    tunnel: [w42] -> w22
    tunnel: [w41] -> w21
    tunnel: [w40] -> w19
    tunnel: [w39] -> w17
    tunnel: [w38] -> w16
    tunnel: ["1D fits?"] -> w15
    tunnel: [w36] -> w13
    tunnel: [w35] -> w12
    tunnel: ["Root Directory"] -> w11
    tunnel: ["Base Filename"] -> w9
    tunnel: ["Load File Names\nFrom Batch File?"] -> w6
    tunnel: [w29] -> w5
    tunnel: ["Load File Names\nFrom Batch File?"] -> w2
    tunnel: [w26] -> w1
    tunnel: w25 -> [w156]
    tunnel: w24 -> [w206]
    tunnel: w23 -> [w205]
    tunnel: w22 -> [w204]
    tunnel: w21 -> [w203]
    tunnel: [w202] -> w20
    tunnel: w19 -> [w202]
    tunnel: [w201] -> w18
    tunnel: w17 -> [w201]
    tunnel: w16 -> [w200]
    tunnel: w15 -> [w198]
    tunnel: [w198] -> w14
    tunnel: w13 -> [w161]
    tunnel: w12 -> [w162]
    tunnel: w11 -> [w170]
    tunnel: [w170] -> w10
    tunnel: w9 -> [w160]
    tunnel: [w160] -> w8
    tunnel: [w159] -> w7
    tunnel: w6 -> [w159]
    tunnel: w5 -> [w158]
    tunnel: [w158] -> w4
    tunnel: [w157] -> w3
    tunnel: w2 -> [w157]
    tunnel: w1 -> [w155]
    tunnel: w20 -> [w263]
    tunnel: w18 -> [w259]
    tunnel: w14 -> [w255]
    tunnel: w10 -> [w254]
    tunnel: w8 -> [w253]
    tunnel: w7 -> [_]
    tunnel: w4 -> [w252]
    tunnel: w3 -> [w249]
    frame #0 {
      # "This Boolean activates 1D fitting."
      # "This frames sends data to\nimage_analysis_bkgnd AND/OR\nMeaghan's 2D fitting routine\nto get fit parameters."
      n2 = case shown="True" "Load File Names\nFrom Batch File?" {
        tunnel: ["Image File List" w52] -> w33
        tunnel: ["Background File List" w53] -> w32
        tunnel: "Root Directory" -> [_ w51]
        tunnel: "Base Filename" -> [_ w50]
        tunnel: ["Changed\nValue" w49] -> w27
        frame False {
        }
        frame True {
          # "File names and changed\nloaded from batch file."
          n3 = call "load_from_batch.vi"("Base File Path"=w51, "Base Filename"=w50) -> ("atoms array"=w52:string[], "bkgnd array"=w53:string[], "Changed Values"=w49:dbl[])
        }
      }
      "Image File List" <- w33
      "Background File List" <- w32
      n4 = for {
        tunnel: w33 -> [w80] mode=indexing
        tunnel: [w94] -> w42 mode=indexing
        tunnel: [w115] -> w40 mode=indexing
        tunnel: [w121] -> w41 mode=indexing
        tunnel: [w120] -> w44 mode=indexing
        tunnel: [w119] -> w43 mode=indexing
        tunnel: "camera background with no image beam\nIt will be subtracted before the log is taken" -> [w116]
        tunnel: w27 -> [w114] mode=indexing
        tunnel: [w89] -> w39 mode=indexing
        tunnel: [w93] -> w38 mode=indexing
        tunnel: "1D fits?" -> [w92]
        tunnel: [w91] -> w36 mode=indexing
        tunnel: [w90] -> w35 mode=indexing
        tunnel: [w87] -> w34 mode=indexing
        tunnel: "Root Directory" -> [w82]
        tunnel: w32 -> [w75] mode=indexing
        tunnel: [w61] -> w26 mode=indexing
        i -> [w88]
        w117 = 0.0
        # "2D Fitting"
        n5 = Unbundle By Name("Specifics of Fitting Routines") -> ("sampleinterleave"=w107:dbl, "pixelsize"=w77:dbl, "CCD Binning"=w78:dbl, "cutborders"=w106:dbl, "numberforscale"=w105:dbl, "limit"=w104:dbl, "guesssmoothsize"=w103:dbl)
        n6 = Path To String(path=w82) -> (string=w86:string)
        n7 = Multiply(x=w77, y=w78) -> (x*y=w60:dbl)
        n8 = Index Array(array="saved image dimensions", index #1=0 ("index"), index #2=1 ("index")) -> (element #1=w68:i32, element #2=w67:i32)
        n9 = Concatenate Strings(w86, "\\", w80) -> (w85:string)
        n10 = Unbundle("Software Binning") -> ("Software\nBinning?"=w58:bool, "Software Bin Size"=w55:i32)
        n11 = String To Path(string=w85) -> (path=w73:path)
        n12 = call "binningsize.vi"("CCD Binning"=w60, "Software Binning"="Software Binning") -> ("Software Bin Size"=w54:i32, "Binning Value"=w59:dbl)
        n13 = Path To String(path=w82) -> (string=w83:string)
        n14 = Concatenate Strings(w83, "\\", w75) -> (w84:string)
        n15 = String To Path(string=w84) -> (path=w72:path)
        n16 = case shown="True" "Read\nBinary?" {
          tunnel: w73 -> [w138 w144]
          tunnel: [w137 w143] -> w63
          tunnel: w72 -> [w136 w141]
          tunnel: [w135 w142] -> w56
          tunnel: w67 -> [_ w139]
          tunnel: w68 -> [_ w140]
          frame False {
            n17 = call-poly <vilib>:"Read From Spreadsheet File.vi"("file path (dialog if empty)"=w138) -> ("all rows"=w137:dbl[][])  [unwired: 6 in, 4 out]
            n18 = call-poly <vilib>:"Read From Spreadsheet File.vi"("file path (dialog if empty)"=w136) -> ("all rows"=w135:dbl[][])  [unwired: 6 in, 4 out]
          }
          frame True {
            n19 = call <vilib>:"Read From I16 File.vi"("2D number of columns/1D count (all as 1D:-1)"=w139, "2D number of rows"=w140, "file path (dialog if empty)"=w144) -> ("2D array"=w143:i16[][])  [unwired: 4 in, 4 out]
            n20 = call <vilib>:"Read From I16 File.vi"("2D number of columns/1D count (all as 1D:-1)"=w139, "2D number of rows"=w140, "file path (dialog if empty)"=w141) -> ("2D array"=w142:i16[][])  [unwired: 4 in, 4 out]
          }
        }
        n21 = call "software_roi.vi"("Cut image?"="Cut image?", "Input Array"=w63, "ROI Controls"="ROI Controls") -> ("output array"=w64:sgl[][])
        n22 = call "software_roi.vi"("Cut image?"="Cut image?", "Input Array"=w56, "ROI Controls"="ROI Controls") -> ("output array"=w66:sgl[][])
        n23 = call "software_binning.vi"("Bin image?"=w58, "Input Array"=w64, "bin size"=w55) -> ("Binned Array"=w62:dbl[][])
        n24 = call "software_binning.vi"("Bin image?"=w58, "Input Array"=w66, "bin size"=w55) -> ("Binned Array"=w65:dbl[][])
        n25 = call "onthefly2DfitR4.vi"("Detuning in MHz"="Image beam \nDetuning (MHz)", "Wavelength (m)"="Wavelength (m)", "pass image method"=TRUE, "Natural Linewidth of Transition\n(ion fwhm in MHz)"="Natural Linewidth of Transition\n(ion fwhm in MHz)", "Scale Base Level?"="scale base level?", "Atoms"=w62, "Background"=w65, "Specifics of Fitting Routines"="Specifics of Fitting Routines", "Software bin size"=w54, "Iteration #"=w88) -> ("2-D Gaussian Fit Parameters"=w87:T6, "peak OD"=w61:dbl, "# atoms from peakOD"=w93:dbl, "Chi-squared"=w96:dbl)  [unwired: 1 in, 5 out]
        n26 = Unbundle By Name(w87) -> ("amplitude"=w102:dbl, "sigma_y (m)"=w91:dbl, "sigma_x (m)"=w90:dbl, "row offset (pixel #)"=w101:dbl, "col offset (pixel #)"=w100:dbl, "offset"=w99:dbl, "slope x"=w98:dbl, "slope y"=w97:dbl)
        n27 = case shown="True" w92 {
          tunnel: [_ w153] -> w134
          tunnel: [_ w152] -> w133
          tunnel: [_ w151] -> w130
          tunnel: w88 -> [_ w150]
          tunnel: w116 -> [_ w149]
          tunnel: w59 -> [_ w148]
          tunnel: w62 -> [_ w147]
          tunnel: w65 -> [_ w145]
          tunnel: "Image beam \nDetuning (MHz)" -> [_ w146]
          frame False {
            # "No 1D\nfitting."
          }
          frame True {
            # "1D Fitting"
            n28 = call "image_analysis_bkgndR3.vi"("Atoms array in"=w147, "BG array in"=w145, "Delta_x (m)"=w148, "Delta_y (m)"=w148, "camera background with no image beam\nIt will be subtracted before the log is taken"=w149, "Image beam \nDetuning (MHz)"=w146, "Iteration #"=w150) -> ("x fit values"=w151:T7, "parameters from \npeak absorption"=w152:T8, "y fit values"=w153:T9)  [unwired: 14 in, 4 out]
          }
        }
        n29 = Bundle("Wavelength (m)"="Wavelength (m)", "Natural Linewidth of Transition\n(ion fwhm in MHz)"="Natural Linewidth of Transition\n(ion fwhm in MHz)", "Image beam \nDetuning (MHz)"="Image beam \nDetuning (MHz)", "sampleinterleave"=w107, "pixelsize"=w77, "cutborders"=w106, "numberforscale"=w105, "limit"=w104, "guesssmoothsize"=w103, "amplitude"=w102, "sigma_y (m)"=w91, "sigma_x (m)"=w90, "row offset (pixel #)"=w101, "col offset (pixel #)"=w100, "offset"=w99, "slope x"=w98, "slope y"=w97, "Chi-squared"=w96, "# atoms from peakOD"=w93) -> (w89:T10)  [unwired: 1 in]
        n30 = Unbundle By Name(w133) -> ("alpha"=w125:dbl, "peakdensity"=w124:dbl, "alphadenssigzsqrt2pi"=w123:sgl, "number"=w122:dbl)
        n31 = Unbundle By Name(w130) -> ("Amplitude"=w132:dbl, "x0"=w131:dbl, "rmswidthx"=w94:dbl, "offsetx"=w129:dbl, "numberx"=w120:dbl)
        n32 = Unbundle By Name(w134) -> ("Amplitude"=w128:dbl, "y0"=w127:dbl, "rmswidthy"=w121:dbl, "offsety"=w126:dbl, "numbery"=w119:dbl)
        n33 = To Double Precision Float(number=w123) -> (double precision float=w118:dbl)
        n34 = Bundle("Numeric"=w114, "Amplitude"=w132, "x0"=w131, "rmswidthx"=w94, "offsetx"=w129, "numberx"=w120, "Amplitude"=w128, "y0"=w127, "rmswidthy"=w121, "offsety"=w126, "numbery"=w119, "alpha"=w125, "peakdensity"=w124, w118, "number"=w122, w117, w117, w117, w117) -> (w115:T11)  [unwired: 1 in]
        "Iteration Number" <- w88
      }
      "1D fits" <- w40
      "2D fits" <- w34
      n35 = Array Size(array=w27) -> (size(s)=w29:i32)
    }
    frame #1 {
      w171 = 0.001
      # "1000*M/Kb"
      # "To correct for millisec"
      # "To correct for millisec"
      # "1000*M/Kb"
      n36 = case shown="True" w198 {
        tunnel: w206 -> [_ w216]
        tunnel: w205 -> [_ w215]
        tunnel: w204 -> [_ w214]
        tunnel: w203 -> [_ w208]
        tunnel: w156 -> [_ w209]
        tunnel: w171 -> [_ w213]
        frame False {
          # "No 1D fitting, thus no 1D plots."
        }
        frame True {
          # "1000*M/Kb"
          # "To correct for millisec"
          # "This frame calculates temperatures\nand sizes from the fit parameters."
          # "1000*M/Kb"
          # "sigma^2=sigma0^2+(KB*T/M) t^2"
          # "To correct for millisec"
          n37 = Bundle("Changed Values"=w209, w215) -> (w219:cluster{"Changed Values":dbl[], dbl[]})  [unwired: 1 in]
          n38 = Bundle("Changed Values"=w209, w216) -> (w218:cluster{"Changed Values":dbl[], dbl[]})  [unwired: 1 in]
          n39 = Build Array(w218, w219) -> (→"Number":cluster{"Changed Values":dbl[], dbl[]}[])
          n40 = Multiply(x=w209, y=w213) -> (x*y=w210:dbl[])
          n41 = Bundle("Changed Values"=w209, w208) -> (w245:cluster{"Changed Values":dbl[], dbl[]})  [unwired: 1 in]
          n42 = Multiply(x=w210, y=w210) -> (x*y=w229:dbl[])
          n43 = Bundle("Changed Values"=w209, w214) -> (w242:cluster{"Changed Values":dbl[], dbl[]})  [unwired: 1 in]
          n44 = Multiply(x=w209, y=w213) -> (x*y=w212:dbl[])
          n45 = Multiply(x=w214, y=w214) -> (x*y=w228:dbl[])
          n46 = Multiply(x=w212, y=w212) -> (x*y=w211:dbl[])
          n47 = Multiply(x=w208, y=w208) -> (x*y=w221:dbl[])
          n48 = call <vilib>:"Linear Fit.vi"("Y"=w228, "X"=w229) -> ("slope"=w207:dbl, "intercept"=w231:dbl)  [unwired: 9 in, 3 out]
          n49 = Square Root(x=w207) -> (sqrt(x)=→"sqrt(KT/M) x":dbl)
          n50 = Square Root(x=w231) -> (sqrt(x)=→"initial size x":dbl)
          n51 = call <vilib>:"Linear Fit.vi"("Y"=w221, "X"=w211) -> ("slope"=w238:dbl, "intercept"=w223:dbl, "residue"=→"mean square error":dbl)  [unwired: 9 in, 2 out]
          n52 = Square Root(x=w223) -> (sqrt(x)=→"initial size Y":dbl)
          n53 = Square Root(x=w238) -> (sqrt(x)=→"sqrt(KT/M) Y":dbl)
          n54 = Multiply(x=w207, y=w229) -> (x*y=w230:dbl[])
          n55 = Multiply(x=w207, y=10.65) -> (x*y=→"Temperature (mK) X":dbl)
          n56 = Add(x=w230, y=w231) -> (x+y=w232:dbl[])
          n57 = Multiply(x=w238, y=w211) -> (x*y=w222:dbl[])
          n58 = Multiply(x=w238, y=10.65) -> (x*y=→"Temperature (mK) Y":dbl)
          n59 = Square Root(x=w232) -> (sqrt(x)=w233:dbl[])
          n60 = Add(x=w222, y=w223) -> (x+y=w224:dbl[])
          n61 = Build Array(w242, w245) -> (→"RMS width":cluster{"Changed Values":dbl[], dbl[]}[])
          n62 = Square Root(x=w224) -> (sqrt(x)=w225:dbl[])
          n63 = Bundle("Changed Values"=w209, w233) -> (w241:cluster{"Changed Values":dbl[], dbl[]})  [unwired: 1 in]
          n64 = Build Array(w241, w242) -> (→"RMS width fitx":cluster{"Changed Values":dbl[], dbl[]}[])
          n65 = Bundle("Changed Values"=w209, w225) -> (w246:cluster{"Changed Values":dbl[], dbl[]})  [unwired: 1 in]
          n66 = Build Array(w246, w245) -> (→"RMS width fity":cluster{"Changed Values":dbl[], dbl[]}[])
        }
      }
      n67 = Multiply(x=w156, y=w171) -> (x*y=w163:dbl[])
      n68 = Bundle("Changed Values"=w156, w200) -> (→"Number Graph":cluster{"Changed Values":dbl[], dbl[]})  [unwired: 1 in]
      n69 = Bundle("Changed Values"=w156, w162) -> (w165:cluster{"Changed Values":dbl[], dbl[]})  [unwired: 1 in]
      n70 = Bundle("Changed Values"=w156, w161) -> (w168:cluster{"Changed Values":dbl[], dbl[]})  [unwired: 1 in]
      n71 = Multiply(x=w161, y=w161) -> (x*y=w196:dbl[])
      n72 = Multiply(x=w163, y=w163) -> (x*y=w195:dbl[])
      n73 = Multiply(x=w156, y=w171) -> (x*y=w183:dbl[])
      n74 = Build Array(w165, w168) -> (→"RMS Widths Graph":cluster{"Changed Values":dbl[], dbl[]}[])
      n75 = call <vilib>:"Linear Fit.vi"("Y"=w196, "X"=w195) -> ("slope"=w189:dbl, "intercept"=w191:dbl, "residue"=w187:dbl)  [unwired: 9 in, 2 out]
      n76 = Multiply(x=w162, y=w162) -> (x*y=w184:dbl[])
      n77 = Multiply(x=w183, y=w183) -> (x*y=w182:dbl[])
      n78 = Multiply(x=w189, y=w195) -> (x*y=w194:dbl[])
      n79 = call <vilib>:"Linear Fit.vi"("Y"=w184, "X"=w182) -> ("slope"=w174:dbl, "intercept"=w178:dbl, "residue"=w176:dbl)  [unwired: 9 in, 2 out]
      n80 = Multiply(x=w174, y=w182) -> (x*y=w181:dbl[])
      n81 = Add(x=w194, y=w191) -> (x+y=w193:dbl[])
      n82 = Multiply(x=10.65 ("y"), y=w189) -> (x*y=→"Temperature (mK) y":dbl)
      n83 = Square Root(x=w193) -> (sqrt(x)=w192:dbl[])
      n84 = Square Root(x=w191) -> (sqrt(x)=→"Initial Size y 2D Fit":dbl)
      n85 = Square Root(x=w187) -> (sqrt(x)=→"Mean Square \nError y 2D Fit":dbl)
      n86 = Bundle("Changed Values"=w156, w192) -> (w169:cluster{"Changed Values":dbl[], dbl[]})  [unwired: 1 in]
      n87 = Add(x=w181, y=w178) -> (x+y=w180:dbl[])
      n88 = Multiply(x=10.65 ("y"), y=w174) -> (x*y=→"Temperature (mK) x":dbl)
      n89 = Square Root(x=w180) -> (sqrt(x)=w179:dbl[])
      n90 = Square Root(x=w178) -> (sqrt(x)=→"Initial Size x 2D Fit":dbl)
      n91 = Square Root(x=w176) -> (sqrt(x)=→"Mean Square\nError x 2D Fit":dbl)
      n92 = Build Array(w168, w169) -> (→"RMS Width Y 2D Fit":cluster{"Changed Values":dbl[], dbl[]}[])
      n93 = Bundle("Changed Values"=w156, w179) -> (w166:cluster{"Changed Values":dbl[], dbl[]})  [unwired: 1 in]
      n94 = Build Array(w165, w166) -> (→"RMS Width X 2D Fit":cluster{"Changed Values":dbl[], dbl[]}[])
      n95 = Bundle("Changed Values"=w156, w155) -> (→"Peak OD versus delay":cluster{"Changed Values":dbl[], dbl[]})  [unwired: 1 in]
    }
    frame #2 {
      n96 = Concatenate Strings(w253, "2Dimages.fit" ("Substring")) -> (w258:string)
      n97 = Concatenate Strings(w253, "images.fit" ("Substring")) -> (w262:string)
      n98 = Not(x=w249) -> (.not. x?=w248:bool)
      n99 = Build Path(base path=w254, name or relative path=w258) -> (appended path=w256:path)
      n100 = Build Path(base path=w254, name or relative path=w262) -> (appended path=w260:path)
      n101 = Or(x=w248, y="Overwrite existing image.fit files on \nstand-alone delayimageanalyse run?") -> (x .or. y?=w251:bool)
      n102 = case shown="True" w251 {
        tunnel: "Array of 6713\nValues" -> [_ w271]
        tunnel: w263 -> [_ w270]
        tunnel: w260 -> [_ w269]
        tunnel: w259 -> [_ w268]
        tunnel: w256 -> [_ w267]
        tunnel: w255 -> [_ w266]
        tunnel: w252 -> [_ w265]
        frame False {
          # "Do not save .images files when re-running analysis."
        }
        frame True {
          n103 = for {
            N: w265 -> [_]
            tunnel: w271 -> [w313] mode=indexing
            tunnel: w270 -> [w315] mode=indexing
            tunnel: w269 -> [w314]
            tunnel: w268 -> [w312] mode=indexing
            tunnel: w267 -> [w311]
            tunnel: w266 -> [w276]
            i -> [w274]
            # "If this is first time in loop,\nwe create new file (or\noverwrite old one).  Else,\nwe append to the existing\nfile."
            # "2dimages.fit file contains the following:\n6713 Array Values\n1-9)\nFitting Controls or Constants\n10) Wavelength\n11) Natural Linewidth\n12) Image Beam Detuning\n13) Sample Interleave (software binning)\n14) Pixel Size\n15) Cut Borders Parameter\n16) Number for Base Scaling\n17) Limit\n18) Smoothing Size\nFit Parameters\n19) Amplitude\n20) Sigma_x\n21) Sigma_y\n22) x offset\n23) y offset\n24) Offset\n25) Slope x\n26) Slope y\n27) Chi-squared value\n28) Number of atoms"
            # "Save 2D fit parameters"
            # "This frame saves 1D and 2D fit parameters\nto \"basefilenameimages.fit\" and\n\"basefilename2Dimages.fit\" files."
            n104 = Array To Cluster(array=w313) -> (cluster=w316:T12)
            n105 = Array To Cluster(array=w313) -> (cluster=w310:T12)
            n106 = Unbundle(w316) -> ("Array of 6713\nValues[0]"=w325:dbl, "Array of 6713\nValues[1]"=w324:dbl, "Array of 6713\nValues[2]"=w323:dbl, "Array of 6713\nValues[3]"=w322:dbl, "Array of 6713\nValues[4]"=w321:dbl, "Array of 6713\nValues[5]"=w320:dbl, "Array of 6713\nValues[6]"=w319:dbl, "Array of 6713\nValues[8]"=w318:dbl)  [unwired: 1 out]
            n107 = Unbundle(w315) -> ("Numeric"=w328:dbl, "Amplitude"=w329:dbl, "x0"=w330:dbl, "rmswidthx"=w331:dbl, "offsetx"=w332:dbl, "numberx"=w333:dbl, "Amplitude"=w334:dbl, "y0"=w335:dbl, "rmswidthy"=w336:dbl, "offsety"=w337:dbl, "numbery"=w338:dbl, "alpha"=w339:dbl, "peakdensity"=w340:dbl, w342:dbl, "number"=w341:dbl)  [unwired: 4 out]
            n108 = To Double Precision Float(number=w342) -> (double precision float=w327:dbl)
            n109 = Unbundle(w310) -> ("Array of 6713\nValues[0]"=w309:dbl, "Array of 6713\nValues[1]"=w308:dbl, "Array of 6713\nValues[2]"=w307:dbl, "Array of 6713\nValues[3]"=w306:dbl, "Array of 6713\nValues[4]"=w305:dbl, "Array of 6713\nValues[5]"=w304:dbl, "Array of 6713\nValues[6]"=w303:dbl, "Array of 6713\nValues[7]"=w302:dbl, "Array of 6713\nValues[8]"=w301:dbl)
            n110 = Unbundle(w312) -> ("Wavelength (m)"=w300:dbl, "Natural Linewidth of Transition\n(ion fwhm in MHz)"=w299:dbl, "Image beam \nDetuning (MHz)"=w298:dbl, "sampleinterleave"=w297:dbl, "pixelsize"=w296:dbl, "cutborders"=w295:dbl, "numberforscale"=w294:dbl, "limit"=w293:dbl, "guesssmoothsize"=w292:dbl, "amplitude"=w291:dbl, "sigma_y (m)"=w290:dbl, "sigma_x (m)"=w289:dbl, "row offset (pixel #)"=w288:dbl, "col offset (pixel #)"=w287:dbl, "offset"=w286:dbl, "slope x"=w285:dbl, "slope y"=w284:dbl, "Chi-squared"=w283:dbl, "# atoms from peakOD"=w282:dbl)
            n111 = Bundle("fmot"="fmot", "Array of 6713\nValues[0]"=w325, "Array of 6713\nValues[1]"=w324, "Array of 6713\nValues[2]"=w323, "Array of 6713\nValues[3]"=w322, "Array of 6713\nValues[4]"=w321, "Array of 6713\nValues[5]"=w320, "Array of 6713\nValues[6]"=w319, "Array of 6713\nValues[8]"=w318, "Numeric"=w328, "Amplitude"=w329, "x0"=w330, "rmswidthx"=w331, "offsetx"=w332, "numberx"=w333, "Amplitude"=w334, "y0"=w335, "rmswidthy"=w336, "offsety"=w337, "numbery"=w338, "alpha"=w339, "peakdensity"=w340, w327, "number"=w341) -> (w326:T13)  [unwired: 1 in]
            n112 = Bundle("Array of 6713\nValues[0]"=w309, "Array of 6713\nValues[1]"=w308, "Array of 6713\nValues[2]"=w307, "Array of 6713\nValues[3]"=w306, "Array of 6713\nValues[4]"=w305, "Array of 6713\nValues[5]"=w304, "Array of 6713\nValues[6]"=w303, "Array of 6713\nValues[7]"=w302, "Array of 6713\nValues[8]"=w301, "Wavelength (m)"=w300, "Natural Linewidth of Transition\n(ion fwhm in MHz)"=w299, "Image beam \nDetuning (MHz)"=w298, "sampleinterleave"=w297, "pixelsize"=w296, "cutborders"=w295, "numberforscale"=w294, "limit"=w293, "guesssmoothsize"=w292, "amplitude"=w291, "sigma_y (m)"=w290, "sigma_x (m)"=w289, "row offset (pixel #)"=w288, "col offset (pixel #)"=w287, "offset"=w286, "slope x"=w285, "slope y"=w284, "Chi-squared"=w283, "# atoms from peakOD"=w282) -> (w277:T14)  [unwired: 1 in]
            n113 = Equal?(x=0, y=w274) -> (x = y?=w273:bool)
            n114 = Cluster To Array(cluster=w277) -> (array=w281:dbl[])
            n115 = case shown="False" w273 {
              tunnel: [TRUE ("append to file? (new file:F)") FALSE ("append to file? (new file:F)")] -> w272
              frame False {
              }
              frame True {
              }
            }
            n116 = case shown="True" w276 {
              tunnel: w326 -> [_ w347]
              tunnel: w314 -> [_ w346]
              tunnel: w272 -> [_ w345]
              frame False {
                # "1D fitting turned off,\nso no saving 1D fit\nparameters."
              }
              frame True {
                # "Save 1D fit parameters"
                n117 = Cluster To Array(cluster=w347) -> (array=w351:dbl[])
                n118 = Array To Spreadsheet String(delimiter (Tab)="\t", array=w351, 3:"%.5e" ("format string")) -> (spreadsheet string=w350:string)
                n119 = call <vilib>:"Write Characters To File.vi"("append to file? (new file:F)"=w345, "character string"=w350, "file path (dialog if empty)"=w346) -> ()  [unwired: 2 in, 1 out]
              }
            }
            n120 = Array To Spreadsheet String(delimiter (Tab)="\t", array=w281, 3:"%.5e" ("format string")) -> (spreadsheet string=w280:string)
            n121 = call <vilib>:"Write Characters To File.vi"("append to file? (new file:F)"=w272, "character string"=w280, "file path (dialog if empty)"=w311) -> ()  [unwired: 2 in, 1 out]
          }
        }
      }
    }
  }
